vi "Report Core.vi"(8 "error in":errorcluster, 9 "Received":path, 10 "Approved":path, 11 "Report With First Working in":refnum<class "Report With First Working.lvclass">) -> (0 "error out":errorcluster, 2 "Worked?":bool, 3 "Report With First Working out":refnum<class "Report With First Working.lvclass">)   [LabVIEW 2020, in "Approval Tests.lvlib" / "Report With First Working.lvclass"]
uses:
  Report With First Working.lvclass
  Report With First Working.lvclass/Report With First Working.ctl
  Reporter/Reporter.lvclass
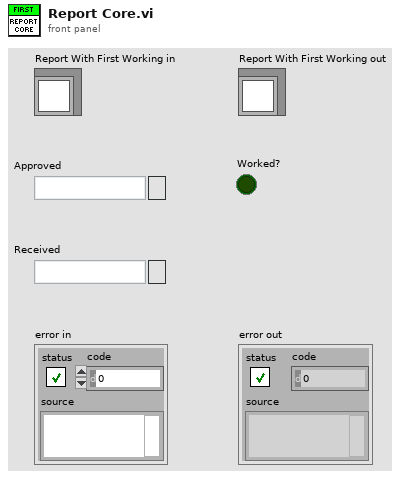
[diagram p1: front panel]
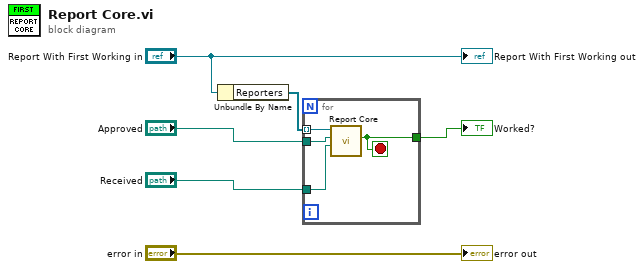
[diagram p0: block diagram]
diagram:
  n1 = Unbundle By Name("Report With First Working in") -> ("Reporters"=w4:refnum<class "Reporter.lvclass">[])
  n2 = for {
    tunnel: w4 -> [w10] mode=indexing
    tunnel: "Approved" -> [w9]
    tunnel: "Received" -> [w8]
    tunnel: [w7] -> w1
    stop <- w7 stop-if-true
    n3 = call-dynamic "Report Core.vi"("Received"=w8, "Approved"=w9, "Reporter in"=w10) -> ("Worked?"=w7:bool)  [unwired: 6 in, 2 out]
  }
  "Worked?" <- w1
  "error out" <- "error in"
  "Report With First Working out" <- "Report With First Working in"
